vi "CombinedHeatPowerUnit.vi"(5 "Day of Year":u32, 6 "Unique Object Identifier":string, 7 "Day Time":u32, 8 "Error In":errorcluster, 10 "Energy flow IN":T6, 11 "DataFlowIN":T5) -> (0 "Error Out":errorcluster, 2 "Energy flow OUT":T6, 3 "DataFlowOUT":T5)   [LabVIEW 2017]
uses:
  classes/DataCollector.lvclass
  classes/DataHandler.lvclass
  classes/SimulationParameter.lvclass
panel:
  out "output cluster":T1
  out "Simulation Parameter":T2
  in  "Operating Parameter":T3
  out "Control Parameter":T4
  out "List of Fieldelements":string[](array[string])
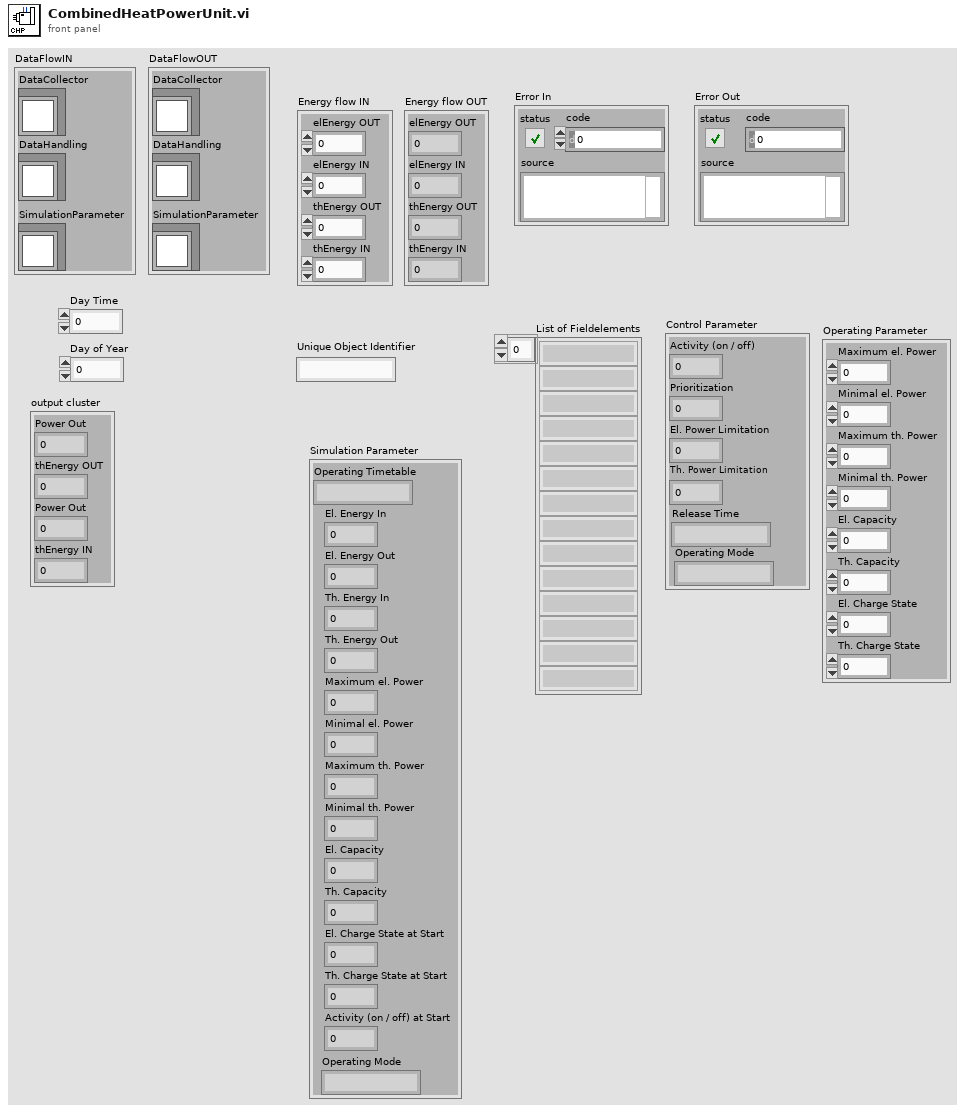
[diagram p1: front panel]
types:
  T1 = cluster{"Power Out":dbl, "thEnergy OUT":dbl, "Power Out":dbl, "thEnergy IN":dbl}
  T2 = cluster{"Operating Timetable":string, "El. Energy In":dbl, "El. Energy Out":dbl, "Th. Energy In":dbl, "Th. Energy Out":dbl, "Maximum el. Power":dbl, "Minimal el. Power":dbl, "Maximum th. Power":dbl, "Minimal th. Power":dbl, "El. Capacity":dbl, "Th. Capacity":dbl, "El. Charge State at Start":dbl, "Th. Charge State at Start":dbl, "Activity (on / off) at Start":i64, "Operating Mode":string}
  T3 = cluster{"Maximum el. Power":dbl, "Minimal el. Power":dbl, "Maximum th. Power":dbl, "Minimal th. Power":dbl, "El. Capacity":dbl, "Th. Capacity":dbl, "El. Charge State":dbl, "Th. Charge State":dbl}
  T4 = cluster{"Activity (on / off)":i64, "Prioritization":i64, "El. Power Limitation":dbl, "Th. Power Limitation":dbl, "Release Time":string, "Operating Mode":string}
  T5 = cluster{"DataCollector":refnum<class "DataCollector.lvclass">, "DataHandling":refnum<class "DataHandler.lvclass">, "SimulationParameter":refnum<class "SimulationParameter.lvclass">}
  T6 = cluster{"elEnergy OUT":dbl, "elEnergy IN":dbl, "thEnergy OUT":dbl, "thEnergy IN":dbl}
  T7 = cluster{"elEnergy OUT":dbl, "thEnergy OUT":dbl, "thEnergy IN":dbl, "thEnergy IN":dbl}
  T8 = cluster{"Day Time":u32, "Day of Year":u32, cluster{"elEnergy OUT":dbl, "thEnergy OUT":dbl, "thEnergy IN":dbl, "thEnergy IN":dbl}, "Operating Parameter":cluster{"Maximum el. Power":dbl, "Minimal el. Power":dbl, "Maximum th. Power":dbl, "Minimal th. Power":dbl, "El. Capacity":dbl, "Th. Capacity":dbl, "El. Charge State":dbl, "Th. Charge State":dbl}, "Control Parameter":cluster{"Activity (on / off)":i64, "Prioritization":i64, "El. Power Limitation":dbl, "Th. Power Limitation":dbl, "Release Time":string, "Operating Mode":string}}
  T9 = cluster{"Day Time":u32, "Day of Year":u32, cluster{"Power Out":dbl, "thEnergy OUT":dbl, "Power Out":dbl, "thEnergy IN":dbl}, "Operating Parameter":cluster{"Maximum el. Power":dbl, "Minimal el. Power":dbl, "Maximum th. Power":dbl, "Minimal th. Power":dbl, "El. Capacity":dbl, "Th. Capacity":dbl, "El. Charge State":dbl, "Th. Charge State":dbl}, "Control Parameter":cluster{"Activity (on / off)":i64, "Prioritization":i64, "El. Power Limitation":dbl, "Th. Power Limitation":dbl, "Release Time":string, "Operating Mode":string}}
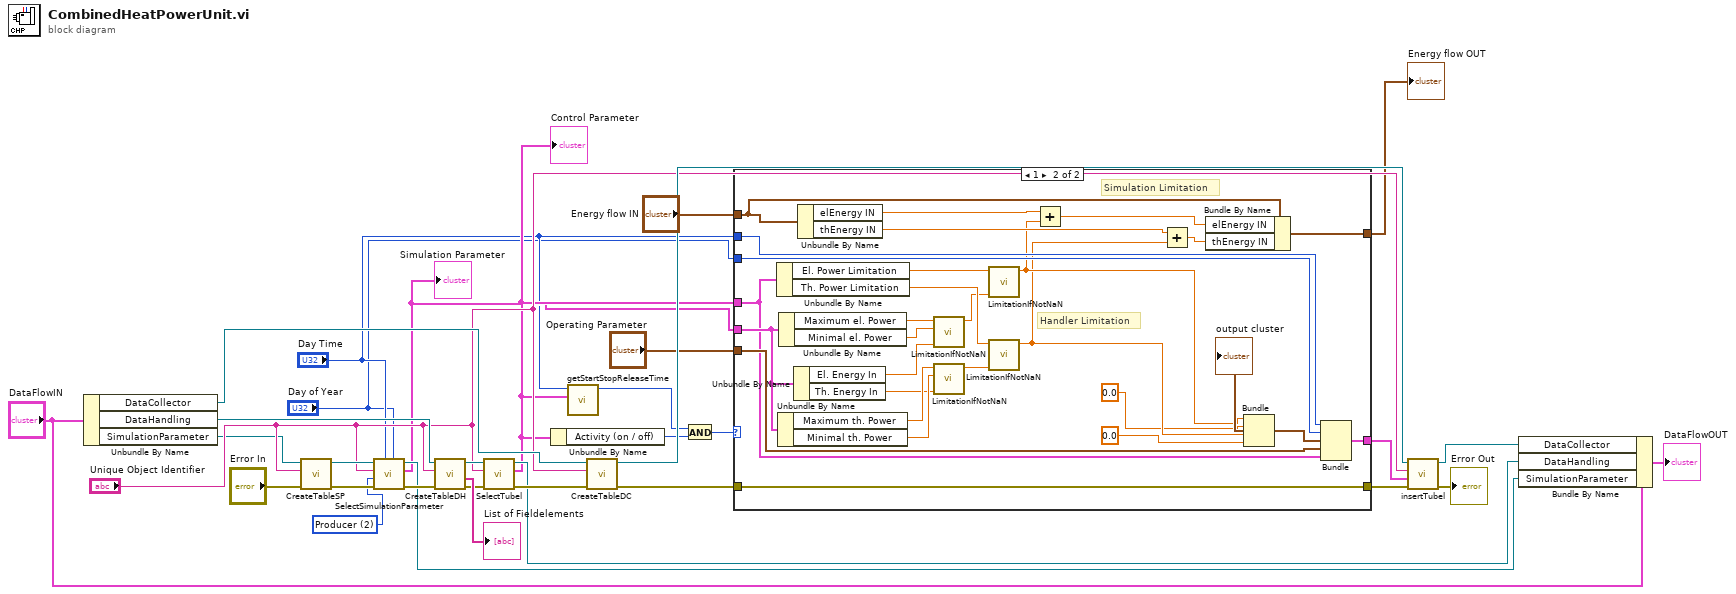
[diagram p0: block diagram]
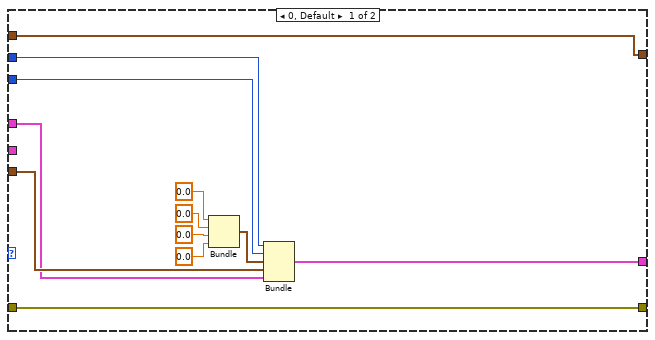
[diagram p2: hidden frame]
diagram:
  w1 = u16 2 items=["External Network", "Consumer", "Producer", "Sorage"] ("Type of Simulation")
  n1 = Unbundle By Name("DataFlowIN") -> ("DataCollector"=w33:refnum<class "DataCollector.lvclass">, "DataHandling"=w23:refnum<class "DataHandler.lvclass">, "SimulationParameter"=w16:refnum<class "SimulationParameter.lvclass">)
  n2 = call-dynamic "CreateTableSP.vi"("error in (no error)"="Error In", "Name of Table"="Unique Object Identifier", "SimulationParameter in"=w16) -> ("error out"=w21:errorcluster, "SimulationParameter out"=w20:refnum<class "SimulationParameter.lvclass">)  [unwired: 5 in, 2 out]
  n3 = call-dynamic "SelectSimulationParameter.vi"("Day of Year"="Day of Year", "Day Time"="Day Time", "error in (no error)"=w21, "Type of Simulation"=w1, "Unique Object Identifier"="Unique Object Identifier", "SimulationParameter in"=w20) -> ("error out"=w18:errorcluster, "Cluster"=w6:T2, "SimulationParameter out"=w15:refnum<class "SimulationParameter.lvclass">)  [unwired: 3 in]
  "Simulation Parameter" <- w6
  n4 = call-dynamic "CreateTableDH.vi"("error in (no error)"=w18, "Name of Table"="Unique Object Identifier", "DataHandler in"=w23) -> ("error out"=w26:errorcluster, "List of Fieldelements"=→"List of Fieldelements":string[], "DataHandler out"=w25:refnum<class "DataHandler.lvclass">)  [unwired: 5 in, 1 out]
  n5 = call-dynamic "SelectTubel.vi"("error in (no error)"=w26, "Unique Object Identifier"="Unique Object Identifier", "DataHandler in"=w25) -> ("error out"=w24:errorcluster, "Control Parameter"=w7:T4, "DataHandler out"=w22:refnum<class "DataHandler.lvclass">)  [unwired: 6 in]
  "Control Parameter" <- w7
  n6 = Unbundle By Name(w7) -> ("Activity (on / off)"=w14:i64)
  n7 = call "getStartStopReleaseTime.vi"("Control Parameter"=w7, "Day Time"="Day Time") -> ("Activity (on / off)"=w12:i64)  [unwired: 9 in]
  n8 = call "CreateTableDC.vi"("error in (no error)"=w24, "Name of Table"="Unique Object Identifier", "DataCollector in"=w33) -> ("error out"=w11:errorcluster, "DataCollector out"=w32:refnum<class "DataCollector.lvclass">)  [unwired: 7 in]
  n9 = And(x=w12, y=w14) -> (x .and. y?=w13:i64)
  n10 = case shown="1" w13 {
    tunnel: w11 -> [w44 w52]
    tunnel: [w44 w52] -> w10
    tunnel: "Day Time" -> [w37 w73]
    tunnel: "Day of Year" -> [w36 w72]
    tunnel: "Operating Parameter" -> [w39 w71]
    tunnel: "Energy flow IN" -> [w45 w68]
    tunnel: [w45 w66] -> w9
    tunnel: w6 -> [_ w67]
    tunnel: w7 -> [w34 w50]
    tunnel: [w35 w51] -> w2
    frame 0, Default {
      n11 = Bundle("elEnergy OUT"=0.0, "thEnergy OUT"=0.0, "thEnergy IN"=0.0, "thEnergy IN"=0.0) -> (w38:T7)  [unwired: 1 in]
      n12 = Bundle("Day Time"=w37, "Day of Year"=w36, w38, "Operating Parameter"=w39, "Control Parameter"=w34) -> (w35:T8)  [unwired: 1 in]
    }
    frame 1 {
      # "Simulation Limitation"
      # "Handler Limitation"
      n13 = Unbundle By Name(w50) -> ("El. Power Limitation"=w58:dbl, "Th. Power Limitation"=w59:dbl)
      n14 = Unbundle By Name(w67) -> ("Maximum th. Power"=w64:dbl, "Minimal th. Power"=w65:dbl)
      n15 = Unbundle By Name(w67) -> ("Maximum el. Power"=w63:dbl, "Minimal el. Power"=w62:dbl)
      n16 = Unbundle By Name(w67) -> ("El. Energy In"=w61:dbl, "Th. Energy In"=w60:dbl)
      n17 = Unbundle By Name(w68) -> ("elEnergy IN"=w70:dbl, "thEnergy IN"=w69:dbl)
      n18 = call "LimitationIfNotNaN.vi"("x"=w61, "Minimal Power"=w62, "Maximum Power"=w63) -> ("Power Out"=w57:dbl)  [unwired: 7 in, 1 out]
      n19 = call "LimitationIfNotNaN.vi"("x"=w60, "Minimal Power"=w65, "Maximum Power"=w64) -> ("Power Out"=w56:dbl)  [unwired: 7 in, 1 out]
      n20 = call "LimitationIfNotNaN.vi"("x"=w57, "Maximum Power"=w58) -> ("Power Out"=w49:dbl)  [unwired: 8 in, 1 out]
      n21 = call "LimitationIfNotNaN.vi"("x"=w56, "Maximum Power"=w59) -> ("Power Out"=w48:dbl)  [unwired: 8 in, 1 out]
      n22 = Add(x=w70, y=w49) -> (x+y=w54:dbl)
      n23 = Add(x=w69, y=w48) -> (x+y=w55:dbl)
      n24 = Bundle By Name(cluster=w68, "elEnergy IN"=w54, "thEnergy IN"=w55) -> (w66:T6)
      n25 = Bundle("Power Out"=w49, "thEnergy OUT"=0.0, "Power Out"=w48, "thEnergy IN"=0.0) -> (w53:T1)  [unwired: 1 in]
      "output cluster" <- w53
      n26 = Bundle("Day Time"=w73, "Day of Year"=w72, w53, "Operating Parameter"=w71, "Control Parameter"=w50) -> (w51:T9)  [unwired: 1 in]
    }
  }
  "Energy flow OUT" <- w9
  n27 = call-dynamic "insertTubel.vi"("error in (no error)"=w10, "Data Cluster"=w2, "Name of Table"="Unique Object Identifier", "DataCollector in"=w32) -> ("error out"=→"Error Out":errorcluster, "DataCollector out"=w31:refnum<class "DataCollector.lvclass">)  [unwired: 6 in]
  n28 = Bundle By Name(cluster="DataFlowIN", "DataCollector"=w31, "DataHandling"=w22, "SimulationParameter"=w15) -> (→"DataFlowOUT":T5)
